vi "Write Cmd.vi"(8 "error in (no error)":errorcluster, 10 "Cmd":string, 11 "PathTokenizer in":refnum<class "PathTokenizer.lvclass">) -> (0 "error out":errorcluster, 3 "PathTokenizer out":refnum<class "PathTokenizer.lvclass">)   [LabVIEW 2019, in "PathTokenizer.lvclass"]
uses:
  PathTokenizer.lvclass
  PathTokenizer.lvclass/PathTokenizer.ctl
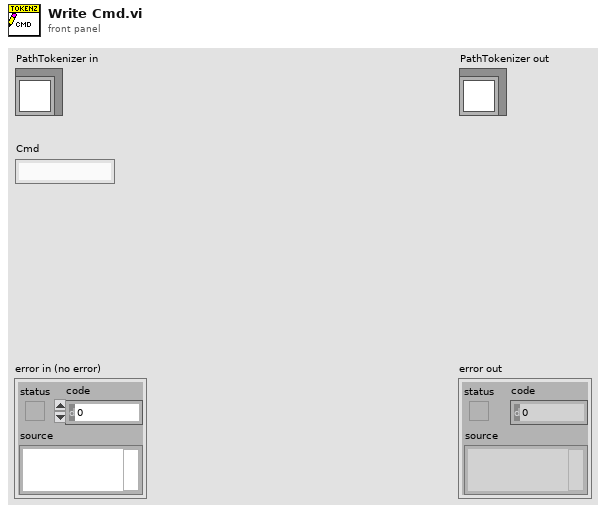
[diagram p1: front panel]
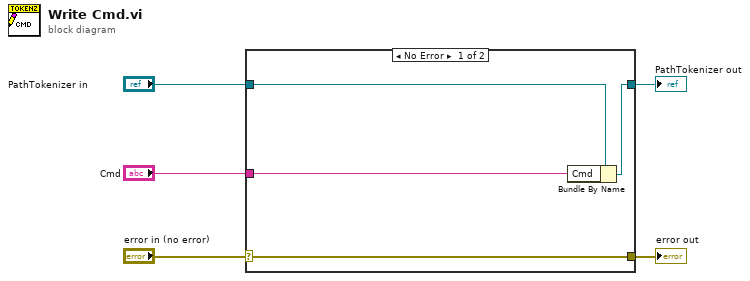
[diagram p0: block diagram]
diagram:
  n1 = case shown="No Error" "error in (no error)" {
    selector: "error in (no error)" -> [w9 w10]
    tunnel: [w9 w10] -> w4
    tunnel: [w7 w11] -> w2
    tunnel: "PathTokenizer in" -> [w8 w11]
    tunnel: "Cmd" -> [w6 _]
    frame No Error {
      n2 = Bundle By Name(cluster=w8, "Cmd"=w6) -> (w7:refnum<class "PathTokenizer.lvclass">)
    }
    frame Error {
    }
  }
  "error out" <- w4
  "PathTokenizer out" <- w2
